vi "HFRR ADV v03.vi"() -> ()   [LabVIEW 2025] (continued)
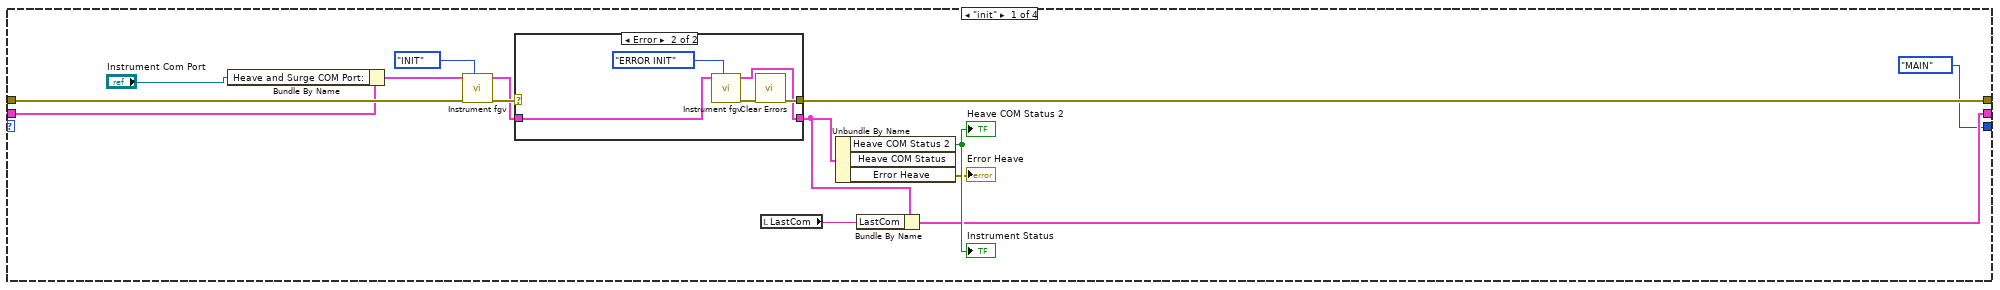
[diagram p2: hidden frame]
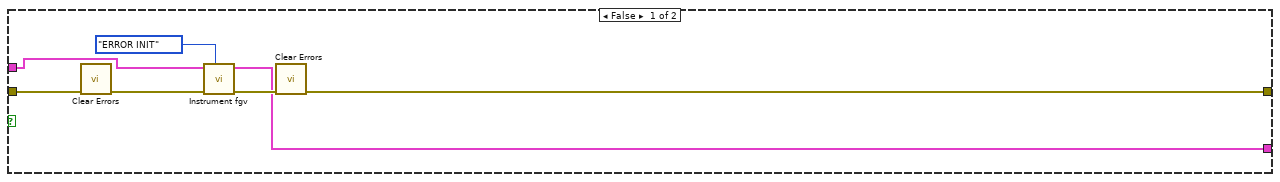
[diagram p4: hidden frame]
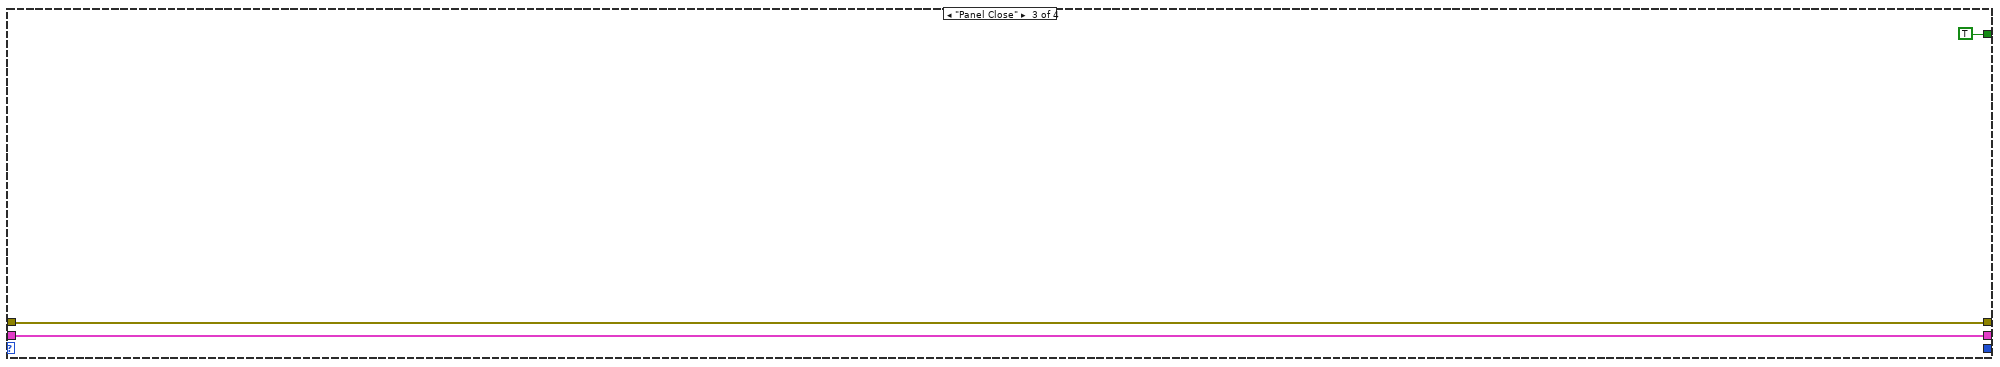
[diagram p8: hidden frame]
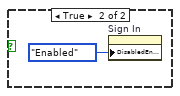
[diagram p19: hidden frame]
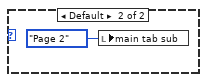
[diagram p20: hidden frame]
            n2897 = Concatenate Strings(w3897, w3906, w3911, w3867) -> (w3870:string)
            n2898 = Concatenate Strings(w3897, w3896, w3905, w3867) -> (w3869:string)
            n2899 = Concatenate Strings(w3897, w3895, w3898, "\"}" ("string")) -> (w3868:string)
            n2900 = Concatenate Strings(w3874, w3873, w3872, w3871, w3870, w3869, w3868, "]}" ("string")) -> (w3865:string)
            n2901 = local read "SEN.RUN HRS"() -> (w3831:dbl)
            n2902 = case shown="True" "Case Constant\n(See Context Help) 3" {
              frame False {
              }
              frame True {
                n2903 = local read "state"() -> (w3951:string[])
                n2904 = Delete From Array(array=w3951, index=0) -> (array with subset deleted=w3949:string[])  [unwired: 1 in, 1 out]
                n2905 = for {
                  N: 6 -> [_]
                  tunnel: w3949 -> [w3962] mode=indexing
                  tunnel: [w3961] -> w3948 mode=indexing
                  n2906 = Equal?(x=w3962, y="Warning") -> (x = y?=w3958:bool)
                  n2907 = Equal?(x=w3962, y="Healthy") -> (x = y?=w3955:bool)
                  n2908 = Select(t="2" ("y"), s=w3958, f="3" ("y")) -> (s? t:f=w3953:string)
                  n2909 = Select(t="1" ("y"), s=w3955, f=w3953) -> (s? t:f=w3961:string)
                }
                "state1" <- w3948
              }
            }
            n2910 = stacked-sequence {
              tunnel: w3865 -> [w3973 _ _]
              tunnel: [_ _ w3989] -> _
              frame #0 {
                (unwired) FALSE ("convert eol (F)")
                w3975 = enum16{"start", "end", "current"}."start" ("pos mode (0:2)")
                n2911 = local read "Path"() -> (w3969:path)
                n2912 = Path To String(path=w3969) -> (string=w3981:string)
                n2913 = Concatenate Strings(w3981, "\\", "Sensor File Name") -> (w3982:string)
                n2914 = local write "standard output 2"(" ") -> ()
                n2915 = String To Path(string=w3982) -> (path=w3972:path)
                n2916 = call <vilib>:"Open_Create_Replace File.vi"("advisory dialog? (display:T)"=FALSE, "function (open:0)"=T19."create or replace", "file path"=w3972) -> ("error out"=w3985:errorcluster, "refnum"=w3984:refnum<file>)  [unwired: 5 in, 2 out]
                n2917 = Set File Position(refnum=w3984, from (0:start)=w3975, error in=w3985) -> (refnum out=w3965:refnum<file>, error out=w3964:errorcluster)  [unwired: 1 in]
                n2918 = Write to Binary File(file (use dialog)=w3965, data=" ", error in=w3964, 5:FALSE ("prepend array or string size? (T)")) -> (refnum out=w3976:refnum<file>, error out=w3977:errorcluster)  [unwired: 2 in, 1 out]
                n2919 = Set File Position(offset (in bytes) (0)=w3975, refnum=w3976, error in=w3977) -> (refnum out=w3968:refnum<file>, error out=w3967:errorcluster)  [unwired: 1 in]
                n2920 = Write to Binary File(file (use dialog)=w3968, data=w3973, error in=w3967, 5:FALSE ("prepend array or string size? (T)")) -> (error out=w3971:errorcluster)  [unwired: 2 in, 2 out]
                n2921 = flat-sequence {
                  tunnel: w3972 -> [w3987]
                  tunnel: w3971 -> [_]
                  frame #0 {
                    n2922 = call <vilib>:"Read Characters From File.vi"("file path (dialog if empty)"=w3987) -> ("character string"=→"Sensor Health JSON string":string)  [unwired: 5 in, 3 out]
                  }
                }
                "SinglePoint  2" <- w3973
              }
              frame #1 {
              }
              frame #2 {
                (unwired) "\"Stored\": true" ("string")
                n2923 = call <vilib>:"System Exec.vi"("run minimized? (F)"=TRUE, "wait until completion? (T)"=TRUE, "working directory"=path "C:/LAB-IQ-NXT", "command line"="C:\\LAB-IQ-NXT\\JPostH.bat") -> ("standard error"=→"Respose From Server 2":string, "standard output"=w3992:string)  [unwired: 4 in, 2 out]
                "standard output 2" <- w3992
                n2924 = Match Pattern(string=w3992, regular expression="JSONH Check String") -> (match substring=w3990:string, offset past match=w3989:i32)  [unwired: 1 in, 2 out]
                n2925 = Equal?(x=w3990, y="JSONH Check String") -> (x = y?=→"Upload \nConfirmed 2":bool)
              }
            }
            n2926 = Divide(x=w3831, y=3600.0 ("f")) -> (x/y=w3824:dbl)
            n2927 = local read "run time"() -> (w3882:string[])
            n2928 = Round To Nearest(number=w3824) -> (nearest integer value=w3823:dbl)
            n2929 = Number To Decimal String(number=w3823) -> (decimal integer string=w3822:string)  [unwired: 1 in]
            n2930 = Index Array(array="Sensor Information", index (col) #1=0 ("disabled index (col)"), index (col) #2=1 ("index (col)"), index (col) #3=2 ("index (col)"), index (col) #4=3 ("index (col)")) -> (element #1=→"Sensor name":string[], element #2=→"model num":string[], element #3=→"run time":string[], element #4=→"state":string[])  [unwired: 4 in]
            n2931 = Insert Into Array(array=w3882, index=1, new element #1=w3822, new element #2=w3822, new element #3=w3822, new element #4=w3822, new element #5=w3822, new element #6=w3822) -> (w3847:string[])
            "run" <- w3847
            n2932 = local read "out"() -> (w3828:string[])
            n2933 = local read "Sensor Information"() -> (w3849:string[][])
            n2934 = Replace Array Subset(array=w3849, new element #1=w3847, index (col) #1=2 ("disabled index (col)"), new element #2=w3828, index (col) #2=3 ("index (col)")) -> (w3848:string[][])  [unwired: 2 in]
            n2935 = local write "Sensor Information"(w3848) -> ()
          }
        }
        n2936 = case shown="True" w3793 {
          frame False {
          }
          frame True {
            n2937 = Equal?(x="FLAG", y=0.0) -> (x = y?=w3804:bool)
            n2938 = case shown="False" w3804 {
              frame False {
                n2939 = Get Date/Time In Seconds() -> (seconds since 1Jan1904=w3810:timestamp)
                n2940 = local read "START 2"() -> (w3808:dbl)
                n2941 = To Double Precision Float(number=w3810) -> (double precision float=w3809:dbl)
                n2942 = Subtract(x=w3809, y=w3808) -> (x-y=→"SENSOR TIME  2":dbl)
              }
              frame True {
                n2943 = Get Date/Time In Seconds() -> (seconds since 1Jan1904=w3812:timestamp)
                n2944 = To Double Precision Float(number=w3812) -> (double precision float=→"START 2":dbl)
                n2945 = local write "FLAG"(100.0 ("FLAG")) -> ()
              }
            }
          }
        }
        n2946 = case shown="True" "Case Constant\n(See Context Help) 2" {
          tunnel: w3797 -> [w3814 w3816]
          tunnel: [w3814 w3815] -> w3796
          frame False {
          }
          frame True {
            n2947 = local read "Json St Flg"() -> (w3817:bool)
            n2948 = case shown="True" w3817 {
              tunnel: w3816 -> [w3818 w3820]
              tunnel: [w3818 w3819] -> w3815
              frame False {
              }
              frame True {
                n2949 = Increment(x=w3820) -> (x+1=w3819:dbl)
                "T cycle" <- w3819
                n2950 = local write "Json St Flg"(FALSE ("Json St Flg")) -> ()
              }
            }
          }
        }
        n2951 = local read "EXIT"() -> (w3790:bool)
      }
    }
  }
  n2952 = stacked-sequence {
    tunnel: [w4191] -> w24
    frame #0 {
      w4191 = FALSE ("Upload \nConfirmed")
      n2953 = local write "Upload \nConfirmed"(w4191) -> ()
      n2954 = local write "St Str"("") -> ()
    }
  }
  n2955 = case shown="True" "Case Constant\n(See Context Help) 4" {
    tunnel: w24 -> [_ w4192]
    frame False {
    }
    frame True {
      n2956 = while {
        tunnel: [w4198] -> _
        tunnel: w4192 -> [_]
        i -> [w4198]
        stop <- w4195 stop-if-true
        n2957 = local read "Json End Flg"() -> (w4197:bool)
        n2958 = Wait (ms)(milliseconds to wait=u32 20 ("Refresh Rate (ms)")) -> ()  [unwired: 1 out]
        n2959 = local read "refresh flag"() -> (w4193:bool)
        n2960 = local read "RUN"() -> (w4194:bool)
        n2961 = And(x=w4194, y=w4193) -> (x .and. y?=w4196:bool)
        n2962 = Or(x=w4196, y=w4197) -> (x .or. y?=w4199:bool)
        "AR Led" <- w4199
        n2963 = case shown="True" w4199 {
          frame False {
          }
          frame True {
            w4216 = "\",\""
            n2964 = local read "UUID"() -> (w4214:string)
            n2965 = local write "refresh flag"(FALSE ("refresh flag")) -> ()
            n2966 = local read "time"() -> (w4203:dbl)
            n2967 = Multiply(x=w4203, y=60.0) -> (x*y=w4202:dbl)
            n2968 = Concatenate Strings("UUID\" : \"", w4214, "\"}") -> (w4217:string)
            n2969 = Number To Fractional String(number=w4202, width (-)=i16 10, precision (6)=i16 4) -> (F-format string=w4231:string)  [unwired: 1 in]
            n2970 = Concatenate Strings("{", "\"Time\":\"", w4231, w4216) -> (w4226:string)
            n2971 = stacked-sequence {
              tunnel: w4216 -> [w4279 w4287 w4294 w4302 w4310 w4319 w4326]
              tunnel: [w4280 _ _ _ _ _ _] -> w4230
              tunnel: [_ w4288 _ _ _ _ _] -> w4229
              tunnel: [_ _ w4295 _ _ _ _] -> w4228
              tunnel: [_ _ _ w4304 _ _ _] -> w4227
              tunnel: w4217 -> [_ _ _ _ _ _ w4337]
              tunnel: [_ _ _ _ _ _ w4336] -> w4213
              tunnel: [_ _ _ _ _ w4316 _] -> w4212
              tunnel: [_ _ _ _ w4309 _ _] -> w4211
              frame #0 {
                n2972 = local read "NORMAL LOAD"() -> (w4278:dbl)
                n2973 = Number To Fractional String(number=w4278, width (-)=i16 10, precision (6)=i16 4) -> (F-format string=w4281:string)  [unwired: 1 in]
                n2974 = Concatenate Strings("NormalLoad\":\"", w4281, w4279) -> (w4280:string)
              }
              frame #1 {
                n2975 = local read "Temp"() -> (w4286:dbl)
                n2976 = Number To Fractional String(number=w4286, width (-)=i16 10, precision (6)=i16 4) -> (F-format string=w4289:string)  [unwired: 1 in]
                n2977 = Concatenate Strings("Temperature\":\"", w4289, w4287) -> (w4288:string)
              }
              frame #2 {
                n2978 = local read "cof"() -> (w4292:dbl)
                n2979 = Number To Fractional String(number=w4292, width (-)=i16 10, precision (6)=i16 4) -> (F-format string=w4296:string)  [unwired: 1 in]
                n2980 = Concatenate Strings("FrictionalForce\":\"", w4296, w4294) -> (w4295:string)
              }
              frame #3 {
                n2981 = local read "Set Hz"() -> (w4300:dbl)
                n2982 = Multiply(x=w4300, y=60.0) -> (x*y=w4299:dbl)
                n2983 = Number To Fractional String(number=w4299, width (-)=i16 10, precision (6)=i16 4) -> (F-format string=w4305:string)  [unwired: 1 in]
                n2984 = Concatenate Strings("Speed\":\"", w4305, w4302) -> (w4304:string)
              }
              frame #4 {
                n2985 = local read "Stroke Ln"() -> (w4308:dbl)
                n2986 = Number To Fractional String(number=w4308, width (-)=i16 10, precision (6)=i16 4) -> (F-format string=w4312:string)  [unwired: 1 in]
                n2987 = Concatenate Strings("LinearDeformation\":\"", w4312, w4310) -> (w4309:string)
              }
              frame #5 {
                n2988 = local read "AIR TEMP"() -> (w4315:dbl)
                n2989 = local read "Json St Flg"() -> (w4317:bool)
                n2990 = local read "Json End Flg"() -> (w4318:bool)
                n2991 = Number To Fractional String(number=w4315, width (-)=i16 10, precision (6)=i16 4) -> (F-format string=w4321:string)  [unwired: 1 in]
                n2992 = Concatenate Strings("Vibration\":\"", w4321, w4319) -> (w4316:string)
                n2993 = And(x=w4317, y=w4318) -> ()  [unwired: 1 out]
              }
              frame #6 {
                n2994 = local read "Json End Flg"() -> (w4325:bool)
                n2995 = Get Date/Time In Seconds() -> (seconds since 1Jan1904=w4333:timestamp)
                n2996 = local read "Json St Flg"() -> (w4324:bool)
                n2997 = To Double Precision Float(number=w4333) -> (double precision float=w4332:dbl)
                n2998 = Subtract(x=w4332, y=2082844800.0) -> (x-y=w4330:dbl)
                n2999 = Number To Fractional String(number=w4330, width (-)=i16 12, precision (6)=i16 0) -> (F-format string=w4327:string)  [unwired: 1 in]
                n3000 = case shown="True" w4325 {
                  tunnel: ["" w4340] -> w4334
                  tunnel: w4327 -> [_ w4341]
                  tunnel: w4326 -> [_ w4339]
                  frame False {
                  }
                  frame True {
                    n3001 = local write "Json End Flg"(FALSE ("Json St Flg")) -> ()
                    n3002 = Concatenate Strings("End\": \"", w4341, w4339) -> (w4340:string)
                  }
                }
                n3003 = case shown="True" w4324 {
                  tunnel: [w4344 w4347] -> w4335
                  tunnel: w4327 -> [_ w4348]
                  tunnel: w4326 -> [_ w4345]
                  frame False {
                    n3004 = local read "St Str"() -> (w4344:string)
                  }
                  frame True {
                    n3005 = Concatenate Strings("Start\":\"", w4348, w4345) -> (w4347:string)
                    "St Str" <- w4347
                    n3006 = local write "Json St Flg"(FALSE ("Json St Flg")) -> ()
                  }
                }
                n3007 = Concatenate Strings(w4335, w4334, w4337) -> (w4336:string)
              }
            }
            n3008 = local read "FILE"() -> (w4205:string)
            n3009 = Concatenate Strings("\",\"OperatorID\":\"" ("string"), "Operator ID") -> (w4208:string)
            n3010 = Concatenate Strings("\",\"DatasetTitle\":\"" ("string"), w4205) -> (w4207:string)
            n3011 = Concatenate Strings("\",\"SerialNumber\":\"" ("string"), "Serial No") -> (w4237:string)
            n3012 = Concatenate Strings("\",\"ModelNumber\":\"" ("string"), "Model No") -> (w4236:string)
            n3013 = Concatenate Strings(w4237, w4236) -> (w4219:string)
            n3014 = Concatenate Strings("{\"SecretKey\":\"", "Secret Key", w4219, w4208, w4207, "\",\"Samples\":[") -> (w4224:string)
            n3015 = Concatenate Strings(w4226, w4230, w4229, w4228, w4227, w4211, w4212, w4213) -> (w4225:string)
            n3016 = Concatenate Strings(w4224, w4225, "]}") -> (w4223:string)
            n3017 = stacked-sequence {
              tunnel: w4223 -> [w4252 _ _]
              tunnel: [_ _ w4269] -> _
              frame #0 {
                (unwired) FALSE ("convert eol (F)")
                w4254 = enum16{"start", "end", "current"}."start" ("pos mode (0:2)")
                n3018 = Path To String(path="Path") -> (string=w4260:string)
                n3019 = Concatenate Strings(w4260, "\\", "Data File Name") -> (w4262:string)
                n3020 = local write "standard output"(" ") -> ()
                n3021 = String To Path(string=w4262) -> (path=w4251:path)
                n3022 = call <vilib>:"Open_Create_Replace File.vi"("advisory dialog? (display:T)"=FALSE, "function (open:0)"=T19."create or replace", "file path"=w4251) -> ("error out"=w4265:errorcluster, "refnum"=w4264:refnum<file>)  [unwired: 5 in, 2 out]
                n3023 = Set File Position(refnum=w4264, from (0:start)=w4254, error in=w4265) -> (refnum out=w4245:refnum<file>, error out=w4244:errorcluster)  [unwired: 1 in]
                n3024 = Write to Binary File(file (use dialog)=w4245, data=" ", error in=w4244, 5:FALSE ("prepend array or string size? (T)")) -> (refnum out=w4255:refnum<file>, error out=w4256:errorcluster)  [unwired: 2 in, 1 out]
                n3025 = Set File Position(offset (in bytes) (0)=w4254, refnum=w4255, error in=w4256) -> (refnum out=w4248:refnum<file>, error out=w4247:errorcluster)  [unwired: 1 in]
                n3026 = Write to Binary File(file (use dialog)=w4248, data=w4252, error in=w4247, 5:FALSE ("prepend array or string size? (T)")) -> (error out=w4250:errorcluster)  [unwired: 2 in, 2 out]
                n3027 = flat-sequence {
                  tunnel: w4251 -> [w4267]
                  tunnel: w4250 -> [_]
                  frame #0 {
                    n3028 = call <vilib>:"Read Characters From File.vi"("file path (dialog if empty)"=w4267) -> ("character string"=→"JSON string":string)  [unwired: 5 in, 3 out]
                  }
                }
                "SinglePoint" <- w4252
              }
              frame #1 {
              }
              frame #2 {
                (unwired) "\"Stored\": true" ("string")
                n3029 = call <vilib>:"System Exec.vi"("run minimized? (F)"=TRUE, "wait until completion? (T)"=TRUE, "working directory"=path "C:/LAB-IQ-NXT", "command line"="C:\\LAB-IQ-NXT\\JPost.bat") -> ("standard error"=→"Respose From Server":string, "standard output"=w4272:string)  [unwired: 4 in, 2 out]
                "standard output" <- w4272
                n3030 = Match Pattern(string=w4272, regular expression="JSON Check String") -> (match substring=w4270:string, offset past match=w4269:i32)  [unwired: 1 in, 2 out]
                n3031 = Equal?(x=w4270, y="JSON Check String") -> (x = y?=→"Upload \nConfirmed":bool)
              }
            }
          }
        }
        n3032 = local read "EXIT"() -> (w4195:bool)
      }
    }
  }
  n3033 = case shown="True" "Case Constant\n(See Context Help) 8" {
    tunnel: w23 -> [_ w4350]
    frame False {
    }
    frame True {
      n3034 = while {
        shift-right: [w4363] -> w4352
        shift-left: _ -> [w4364]
        shift-right: [w4361] -> w4353
        shift-left: errorcluster {"status"=TRUE, "code"=0, "source"="Init"} ("error out") -> [w4362]
        shift-right: [w4359] -> _
        shift-left: "" -> [w4360]
        tunnel: [w4357] -> _
        tunnel: w4350 -> [_]
        i -> [w4357]
        stop <- w4356 stop-if-true
        n3035 = flat-sequence {
          tunnel: [w4365] -> w4358
          frame #0 {
            n3036 = Wait (ms)(milliseconds to wait=10.0 ("Delay")) -> (millisecond timer value=w4365:u32)
          }
        }
        n3037 = case shown="No Error" w4362 {
          selector: w4362 -> [w4398 w4520]
          tunnel: [w4380 w4522] -> w4363
          tunnel: [w4379 w4521] -> w4361
          tunnel: w4364 -> [w4399 w4514]
          tunnel: w4360 -> [w4378 w4513]
          tunnel: [w4377 w4513] -> w4359
          tunnel: w4358 -> [_ _]
          frame No Error {
            n3038 = Concatenate Strings("COMMAND", "\r", "\n") -> (w4389:string)
            n3039 = case shown="True" "Measure" {
              tunnel: w4399 -> [w4425 w4432]
              tunnel: w4398 -> [w4424 w4431]
              tunnel: [w4425 w4430] -> w4397
              tunnel: [w4424 w4429] -> w4376
              tunnel: w4389 -> [_ w4428]
              frame False {
              }
              frame True {
                n3040 = VISA Write(VISA resource name=w4432, write buffer=w4428, error in (no error)=w4431) -> (VISA resource name out=w4430:refnum<visa-resource-name>, error out=w4429:errorcluster)  [unwired: 1 out]
                n3041 = local write "Read String"("") -> ()
                n3042 = local write "Measure"(FALSE) -> ()
              }
            }
            n3043 = property class="Instr"(reference=w4397, error in=w4376) -> (reference out=w4396:refnum<visa-resource-name>, error out=w4395:errorcluster, "Serial Settings:Number of Bytes at Serial Port"=w4394:u32)
            n3044 = Greater?(x=w4394, y=u32 100) -> (0:w4392:bool)
            n3045 = case shown="True" w4392 {
              tunnel: w4396 -> [w4435 w4460]
              tunnel: w4395 -> [w4434 w4459]
              tunnel: w4394 -> [_ w4458]
              tunnel: [w4435 w4457] -> w4382
              tunnel: [w4434 w4456] -> w4381
              tunnel: w4378 -> [w4433 w4455]
              tunnel: [w4433 ""] -> w4377
              frame False {
              }
              frame True {
                w4445 = u32 6 ("y")
                # "Page 84 of \nmanual"
                n3046 = VISA Read(VISA resource name=w4460, byte count=w4458, error in (no error)=w4459) -> (VISA resource name out=w4457:refnum<visa-resource-name>, read buffer=w4453:string, error out=w4456:errorcluster)  [unwired: 1 out]
                n3047 = while {
                  tunnel: w4453 -> [w4509]
                  tunnel: [w4505] -> w4447 mode=indexing
                  tunnel: [w4499] -> w4451 mode=indexing
                  tunnel: [w4497] -> _
                  i -> [w4497]
                  stop <- w4502 stop-if-true
                  n3048 = String Subset(string=w4509, offset (0)=w4497) -> (substring=w4504:string)  [unwired: 1 in]
                  n3049 = String To Byte Array(string=w4504) -> (unsigned byte array=w4508:u8[])
                  n3050 = String Length(string=w4504) -> (length=w4503:i32)
                  n3051 = Index Array(array=w4508) -> (element=w4507:u8)  [unwired: 1 in]
                  n3052 = Equal To 0?(x=w4503) -> (x = 0?=w4502:bool)
                  n3053 = Number To Boolean Array(number=w4507) -> (Boolean array=w4501:bool[])
                  n3054 = Reverse 1D Array(array=w4501) -> (reversed array=w4500:bool[])
                  n3055 = And(x=w4501, y=bool[] [FALSE, FALSE, FALSE, FALSE, FALSE, FALSE, TRUE, TRUE] ("Boolean array")) -> (x .and. y?=w4505:bool[])
                  n3056 = And(x=w4500, y=bool[] [FALSE, FALSE, TRUE, TRUE, TRUE, TRUE, TRUE, TRUE] ("Boolean array")) -> (x .and. y?=w4499:bool[])
                }
                n3057 = Concatenate Strings(w4455, w4453) -> (→"Read String":string)
                n3058 = while {
                  tunnel: w4447 -> [w4496] mode=indexing
                  tunnel: [w4492] -> w4450
                  i -> [w4492]
                  stop <- w4493 stop-if-true
                  n3059 = Search 1D Array(1D array=w4496, element=TRUE) -> (index of element=w4494:i32)  [unwired: 1 in]
                  n3060 = Less Than 0?(x=w4494) -> (x < 0?=w4493:bool)
                }
                n3061 = Delete From Array(array=w4451, length=w4450, index (row)=0) -> (array with subset deleted=w4446:bool[][])  [unwired: 1 in, 1 out]
                n3062 = Array Size(array=w4446) -> (size(s)=w4448:i32[])
                n3063 = Index Array(array=w4448) -> (element=w4440:i32)  [unwired: 1 in]
                n3064 = Greater?(x=w4440, y=w4445) -> (0:w4443:bool)
                n3065 = Subtract(x=w4440, y=w4445) -> (x-y=w4444:u32)
                n3066 = Select(t=w4444, s=w4443, f=u32 0) -> (s? t:f=w4441:u32)
                n3067 = while {
                  tunnel: w4446 -> [w4479]
                  tunnel: [w4481] -> w4439 mode=indexing
                  tunnel: w4441 -> [w4463]
                  i -> [w4480]
                  stop <- w4478 stop-if-true
                  w4470 = 6 ("index")
                  w4469 = 2 ("length")
                  # "Page 65 of \nmanual"
                  n3068 = Multiply(x=u32 3 ("y"), y=w4480) -> (x*y=w4477:u32)
                  n3069 = Divide(x=u32 102 ("y"), y=u32 65520) -> (x/y=w4487:dbl)
                  n3070 = Greater Or Equal?(x=w4477, y=w4463) -> (x >= y?=w4478:bool)
                  n3071 = Index Array(array=w4479, index (row) #1=w4477) -> (element #1=w4475:bool[], element #2=w4474:bool[], element #3=w4473:bool[])  [unwired: 5 in]
                  n3072 = Reverse 1D Array(array=w4475) -> (reversed array=w4468:bool[])
                  n3073 = Reverse 1D Array(array=w4474) -> (reversed array=w4472:bool[])
                  n3074 = Reverse 1D Array(array=w4473) -> (reversed array=w4471:bool[])
                  n3075 = Delete From Array(array=w4468, length=w4469, index=w4470) -> (array with subset deleted=w4464:bool[])  [unwired: 1 out]
                  n3076 = Delete From Array(array=w4472, length=w4469, index=w4470) -> (array with subset deleted=w4465:bool[])  [unwired: 1 out]
                  n3077 = Delete From Array(array=w4471, length=w4469, index=w4470) -> (array with subset deleted=w4466:bool[])  [unwired: 1 out]
                  n3078 = Insert Into Array(array=bool[] [] ("Boolean array"), new element #1=w4464, new element #2=w4465, new element #3=w4466) -> (w4467:bool[])  [unwired: 1 in]
                  n3079 = Boolean Array To Number(Boolean array=w4467) -> (number=w4476:u32)
                  n3080 = Multiply(x=w4487, y=w4476) -> (x*y=w4486:dbl)
                  n3081 = Decrement(x=w4486) -> (x-1=w4485:dbl)
                  n3082 = Divide(x=w4485, y=u32 100) -> (x/y=w4483:dbl)
                  n3083 = Multiply(x=w4483, y=u32 10) -> (x*y=w4481:dbl)
                }
                n3084 = Delete From Array(array=w4439) -> (array with subset deleted=w4438:dbl[])  [unwired: 2 in, 1 out]
                "Waveform Graph 5" <- w4438
                "Waveform Chart 3" <- w4438
                n3085 = call-poly <vilib>:"Mean.vi"("X"=w4438) -> ("mean"=w4437:dbl)  [unwired: 1 out]
                "Measure_LDS" <- w4437
                n3086 = case shown="True" "Zero 4" {
                  tunnel: w4437 -> [_ w4462]
                  frame False {
                  }
                  frame True {
                    n3087 = local write "Zero 4"(FALSE ("Zero 4")) -> ()
                    "z_measure" <- w4462
                  }
                }
              }
            }
            n3088 = local read "Measure_LDS"() -> (w4372:dbl)
            n3089 = local read "Disp (mm)"() -> (w4371:dbl)
            n3090 = local read "Boolean 7"() -> (w4370:bool)
            n3091 = local read "Boolean 8"() -> (w4369:bool)
            n3092 = case shown="True" "Boolean 8" {
              tunnel: w4371 -> [_ w4402]
              tunnel: w4372 -> [_ w4401]
              frame False {
              }
              frame True {
                n3093 = local read "Captured Values 2"() -> (w4405:dbl[][])
                n3094 = Build Array(w4402, w4401) -> (w4400:dbl[])
                n3095 = Build Array (concatenate)(w4405, w4400) -> (w4403:dbl[][])
                n3096 = local write "Captured Values 2"(w4403) -> ()
                n3097 = local write "Boolean 8"(FALSE ("Boolean 8")) -> ()
              }
            }
            n3098 = call "Build XY Graph"("Enable"=w4369, "Reset"=w4370, "Y Input"=w4372, "X Input"=w4371) -> ("XY Graph"=→"?":cluster{"Y":dbl[], "Y":dbl[]}[])  [unwired: 6 in, 1 out]
            n3099 = case shown="True" "Boolean 9" {
              frame False {
              }
              frame True {
                n3100 = local read "Captured Values 2"() -> (w4407:dbl[][])
                n3101 = Index Array(array=w4407, index (col) #1=0 ("disabled index (col)"), index (col) #2=1 ("index (col)")) -> (element #1=w4410:dbl[], element #2=w4409:dbl[])  [unwired: 2 in]
                n3102 = call <vilib>:"Linear Fit.vi"("Y"=w4410, "X"=w4409) -> ("slope"=→"Slope":dbl, "intercept"=→"Intercept":dbl)  [unwired: 9 in, 3 out]
                n3103 = local write "Boolean 9"(FALSE ("Boolean 9")) -> ()
              }
            }
            n3104 = case shown="True" "Boolean 7" {
              frame False {
              }
              frame True {
                n3105 = local write "Captured Values 2"(dbl[][] [] ("Captured Values")) -> ()
                n3106 = local write "Boolean 7"(FALSE ("Boolean 7")) -> ()
              }
            }
            n3107 = Concatenate Strings("COMMAND 2", "\r", "\n") -> (w4384:string)
            n3108 = case shown="True" "Measure 2" {
              tunnel: w4382 -> [w4417 w4423]
              tunnel: w4381 -> [w4416 w4422]
              tunnel: [w4417 w4421] -> w4380
              tunnel: [w4416 w4420] -> w4379
              tunnel: w4384 -> [_ w4419]
              frame False {
              }
              frame True {
                n3109 = local write "Measure 2"(FALSE ("WRITE")) -> ()
                n3110 = VISA Write(VISA resource name=w4423, write buffer=w4419, error in (no error)=w4422) -> (VISA resource name out=w4421:refnum<visa-resource-name>, error out=w4420:errorcluster)  [unwired: 1 out]
              }
            }
          }
          frame Error {
            w4512 = u16 10 items=["1.0"=10, "1.5"=15, "2.0"=20] ("stop bits (10: 1 bit)")
            n3111 = Wait (ms)(milliseconds to wait=u32 20) -> ()  [unwired: 1 out]
            n3112 = VISA Close(VISA resource name=w4514, error in (no error)=w4520) -> (error out=w4519:errorcluster)
            n3113 = call <vilib>:"Clear Errors.vi"("error in (no error)"=w4519) -> ("error out"=w4518:errorcluster)  [unwired: 5 in, 1 out]
            n3114 = call-poly "VISA Configure Serial Port"("VISA resource name"="Laser Disp Sensor", "timeout (10sec)"=u32 200, "Enable Termination\nChar (T)"=TRUE ("Enable Termination\nChar (T)"), "baud rate (9600)"=u32 921600, "error in (no error)"=w4518, "stop bits (10: 1 bit)"=w4512) -> ("VISA resource name out"=w4522:refnum<visa-resource-name>, "error out"=w4521:errorcluster)  [unwired: 8 in]
          }
        }
        n3115 = local read "EXIT"() -> (w4356:bool)
      }
      n3116 = VISA Close(VISA resource name=w4352, error in (no error)=w4353) -> (error out=w4351:errorcluster)
      n3117 = call <vilib>:"Clear Errors.vi"("error in (no error)"=w4351) -> ()  [unwired: 5 in, 2 out]
    }
  }
  n3118 = case shown="True" "Case Constant\n(See Context Help) 9" {
    tunnel: w23 -> [_ w4523]
    frame False {
    }
    frame True {
      n3119 = while {
        tunnel: [w4534] -> _
        shift-right: [w4531] -> w4525
        shift-left: _ -> [w4533]
        shift-right: [w4532] -> w4526
        shift-left: errorcluster {"status"=TRUE, "code"=0, "source"="Init"} ("error out") -> [w4530]
        tunnel: w4523 -> [_]
        i -> [w4534]
        stop <- w4528 stop-if-true
        n3120 = flat-sequence {
          tunnel: w4530 -> [w4625]
          tunnel: [w4625] -> w4529
          frame #0 {
            n3121 = Wait (ms)(milliseconds to wait=u32 50) -> ()  [unwired: 1 out]
          }
        }
        n3122 = case shown="No Error" w4529 {
          selector: w4529 -> [w4575 w4618]
          tunnel: w4533 -> [w4574 w4617]
          tunnel: [w4541 w4608] -> w4532
          tunnel: [w4542 w4616] -> w4531
          frame No Error {
            w4568 = T20 {"Mode"=enum."RTU", "Slave Address"=1} ("Serial Parameters")
            n3123 = call-poly <vilib>:"MB Serial Master Query (poly).vi"("VISA resource name"=w4574, "Starting Address"=i16 1000, "Quantity"=u16 1, "Timeout"=u32 1000, "error in"=w4575, "Serial Parameters"=w4568) -> ("VISA resource name out"=w4569:refnum<visa-resource-name>, "Input Registers"=w4571:u16[], "error out"=w4567:errorcluster)  [unwired: 10 in, 1 out]
            n3124 = Random Number (0-1)() -> (number: 0 to 1=w4556:dbl)
            n3125 = Index Array(array=w4571, index=0) -> (element=w4566:u16)
            n3126 = Subtract(x=w4556, y=0.5) -> (x-y=w4555:dbl)
            n3127 = Divide(x=w4566, y=10 ("index")) -> (x/y=w4560:dbl)
            n3128 = Multiply(x=w4555, y=0.5) -> (x*y=w4554:dbl)
            n3129 = Add(x=w4560, y=w4554) -> (x+y=w4559:dbl)
            n3130 = local read "Amb temp"() -> (w4543:dbl)
            n3131 = Multiply(x=w4559, y=0.2) -> (x*y=w4563:dbl)
            n3132 = Multiply(x=w4543, y=0.8) -> (x*y=w4561:dbl)
            n3133 = Add(x=w4563, y=w4561) -> (x+y=w4544:dbl)
            n3134 = local read "set temp old"() -> (w4538:dbl)
            n3135 = local write "Amb temp"(w4544) -> ()
            n3136 = Select(t="SetTemp 2", s="Heater", f=100.0) -> (s? t:f=w4539:dbl)
            n3137 = Not Equal?(x=w4539, y=w4538) -> (x != y?=w4537:bool)
            n3138 = case shown="True" w4537 {
              tunnel: w4569 -> [w4603 w4605]
              tunnel: [w4602 w4605] -> w4549
              tunnel: w4567 -> [w4601 w4604]
              tunnel: [w4600 w4604] -> w4547
              tunnel: w4539 -> [w4595 _]
              tunnel: w4568 -> [w4597 w4606]
              tunnel: [w4597 w4606] -> w4550
              frame True {
                n3139 = Multiply(x=w4595, y=10 ("index")) -> (x*y=w4594:dbl)
                n3140 = call-poly <vilib>:"MB Serial Master Query (poly).vi"("VISA resource name"=w4603, "Address"=u16 0, "Holding Register"=w4594, "Timeout"=u32 1000, "error in"=w4601, "Serial Parameters"=w4597) -> ("VISA resource name out"=w4602:refnum<visa-resource-name>, "error out"=w4600:errorcluster)  [unwired: 11 in, 1 out]
                "set temp old" <- w4595
              }
              frame False {
              }
            }
            n3141 = flat-sequence {
              tunnel: [w4576] -> _
              tunnel: [w4576] -> w4546
              tunnel: w4547 -> [w4576]
              frame #0 {
                n3142 = Wait (ms)(milliseconds to wait=u32 100) -> ()  [unwired: 1 out]
              }
            }
            n3143 = call "Elapsed Time12"("Time Target (s)"=2.0, "Auto Reset"=TRUE) -> ("Time has Elapsed"=w4551:bool)  [unwired: 10 in, 7 out]
            n3144 = case shown="True" w4551 {
              tunnel: w4550 -> [w4580 w4593]
              tunnel: [w4580 w4593] -> _
              tunnel: [w4579 w4591] -> w4542
              tunnel: w4549 -> [w4579 w4592]
              tunnel: [w4578 w4589] -> w4541
              tunnel: w4546 -> [w4578 w4590]
              frame False {
              }
              frame True {
                n3145 = call-poly <vilib>:"MB Serial Master Query (poly).vi"("VISA resource name"=w4592, "Starting Address"=i16 1003 ("Addr"), "Quantity"=u16 1, "Timeout"=u32 1000, "error in"=w4590, "Serial Parameters"=w4593) -> ("VISA resource name out"=w4591:refnum<visa-resource-name>, "Input Registers"=w4586:u16[], "error out"=w4589:errorcluster)  [unwired: 10 in, 1 out]
                n3146 = Index Array(array=w4586, index=0) -> (element=w4585:u16)
                n3147 = Divide(x=w4585, y=u16 10) -> (x/y=w4581:dbl)
                n3148 = local write "set temp old"(w4581) -> ()
                n3149 = local write "SetTemp"(w4581) -> ()
              }
            }
            "Error Code" <- w4541
            n3150 = Unbundle(w4541) -> ("status"=→"TK4 status":bool)  [unwired: 2 out]
            "SetTemp" <- "SetTemp 2"
          }
          frame Error {
            w4620 = u16 0 items=["None", "Odd", "Even", "Mark", "Space"] ("Parity")
            w4621 = u16 0 items=["None", "XON/XOFF", "RTS/CTS", "XON/XOFF & RTS/CTS", "DTR/DSR", "XON/XOFF & DTR/DSR"] ("Flow Control")
            n3151 = VISA Clear(VISA resource name=w4617, error in (no error)=w4618) -> (VISA resource name out=w4611:refnum<visa-resource-name>, error out=w4609:errorcluster)
            n3152 = VISA Close(VISA resource name=w4611, error in (no error)=w4609) -> (error out=w4610:errorcluster)
            n3153 = call <vilib>:"Clear Errors.vi"("error in (no error)"=w4610) -> ("error out"=w4619:errorcluster)  [unwired: 5 in, 1 out]
            n3154 = Unbundle By Name(T20 {"Mode"=enum."RTU", "Slave Address"=1} ("input cluster")) -> ("Mode"=w4622:enum16{"RTU", "ASCII"})
            n3155 = call <vilib>:"MB Serial Init.vi"("Timeout"=u32 100, "Flow Control"=w4621, "Mode"=w4622, "error in (no error)"=w4619, "Parity"=w4620, "Baud Rate"=u32 9600, "VISA resource name"="Lubrication System COM Port :") -> ("error out"=w4608:errorcluster, "VISA resource name out"=w4616:refnum<visa-resource-name>)  [unwired: 3 in]
            n3156 = local write "set temp old"(0.0 ("set temp old")) -> ()
            n3157 = Unbundle(w4608) -> ("status"=w4607:bool)  [unwired: 2 out]
            n3158 = case shown="True" w4607 {
              selector: w4607 -> [_ w4624]
              frame False {
              }
              frame True {
                n3159 = local write "TK4 status"(w4624) -> ()
              }
            }
          }
        }
        n3160 = local read "EXIT"() -> (w4528:bool)
      }
      n3161 = VISA Close(VISA resource name=w4525, error in (no error)=w4526) -> (error out=w4524:errorcluster)
      n3162 = call <vilib>:"Clear Errors.vi"("error in (no error)"=w4524) -> ()  [unwired: 5 in, 2 out]
    }
  }
  "file count" <- 0 ("file count")
